vi "AddGBSEQ.vi"(0 "VISA resource name":refnum<visa-resource-name>, 1 "Test Current (A)":string, 2 "Dwell Time (s)":string, 3 "Min GB Limit (ohm)":string, 4 "Max GB Limit (ohm)":string, 5 "error in (no error)":errorcluster, 6 "Sequence Number":string, 8 "Sequence Name":string) -> (14 "VISA resource name out":refnum<visa-resource-name>, 17 "Error Message":string, 18 "Error Code":i32, 19 "error out":errorcluster)   [LabVIEW 2010, in "VITREK V7X.lvlib"]
doc: "Add a new GB test step into a sequence and save this sequence into the requested store number."
uses:
  VITREK V7X.lvlib
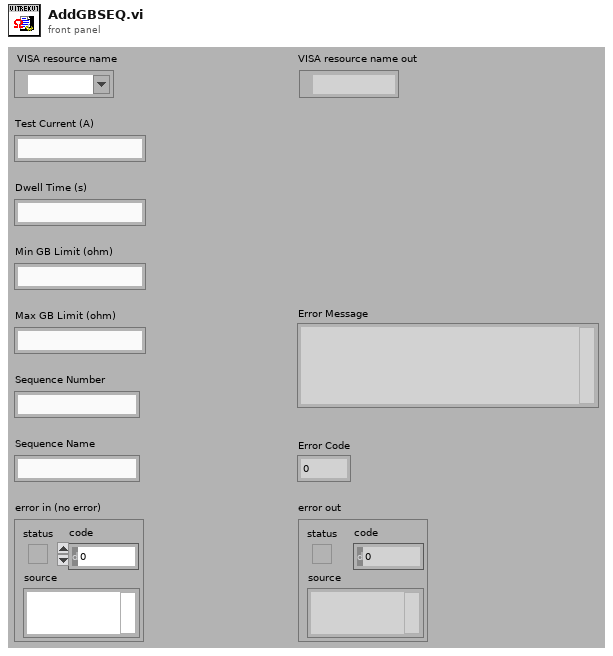
[diagram p1: front panel]
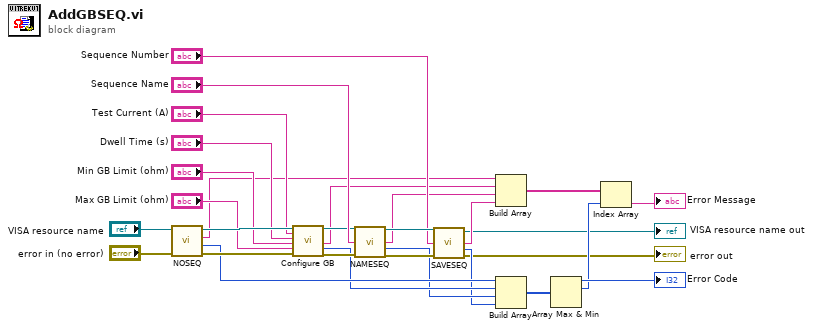
[diagram p0: block diagram]
diagram:
  n1 = call "NOSEQ.vi"("error in (no error)"="error in (no error)", "VISA resource name"="VISA resource name") -> ("error out"=w21:errorcluster, "Error Code"=w11:i32, "Error Message"=w7:string, "VISA resource name out"=w23:refnum<visa-resource-name>)  [unwired: 6 in]
  n2 = call "Configure GB.vi"("VISA resource name"=w23, "Test Current (A)"="Test Current (A)", "Dwell Time (s)"="Dwell Time (s)", "Min GB Limit (ohm)"="Min GB Limit (ohm)", "Max GB Limit (ohm)"="Max GB Limit (ohm)", "error in (no error)"=w21) -> ("VISA resource name out"=w22:refnum<visa-resource-name>, "Error Message"=w6:string, "Error Code"=w10:i32, "error out"=w20:errorcluster)  [unwired: 9 in, 1 out]
  n3 = call "NAMESEQ.vi"("VISA resource name"=w22, "Sequence Name"="Sequence Name", "error in (no error)"=w20) -> ("VISA resource name out"=w26:refnum<visa-resource-name>, "Error Message"=w5:string, "Error Code"=w9:i32, "error out"=w27:errorcluster)  [unwired: 9 in]
  n4 = call "SAVESEQ.vi"("VISA resource name"=w26, "Sequence Number"="Sequence Number", "error in (no error)"=w27) -> ("VISA resource name out"=→"VISA resource name out":refnum<visa-resource-name>, "Error Message"=w4:string, "Error Code"=w8:i32, "error out"=→"error out":errorcluster)  [unwired: 9 in]
  n5 = Build Array(w7, w6, w5, w4) -> (w15:string[])
  n6 = Build Array(w11, w10, w9, w8) -> (w13:i32[])
  n7 = Array Max & Min(array=w13) -> (max value=→"Error Code":i32, max index (indices)=w3:i32)  [unwired: 2 out]
  n8 = Index Array(array=w15, index=w3) -> (element=→"Error Message":string)
